vi "Module Loop.vi"(8 "error in (no error)":errorcluster, 11 "Debug GUI Module in":refnum<class "Debug GUI Module.lvclass">) -> (0 "error out":errorcluster, 3 "Debug GUI Module out":refnum<class "Debug GUI Module.lvclass">)   [LabVIEW 2020, in "VolatusGUI.lvlib" / "Debug GUI Module.lvclass"]
uses:
  Debug GUI Module.lvclass
  C:/dev/lv20CE/relink/lv-volatus/Volatus/Module/Module.lvclass
  Volatus/Module/Module.lvclass/Module.ctl
  Debug GUI Module.lvclass/Debug GUI Module.ctl
  Volatus/Module/Module.lvclass
  Show Module Data.ctl
  Volatus/Module Identity/Module Identity.lvclass/Module Identity.ctl
  Volatus/Show GUI Options.ctl
  Volatus/MessageQ/MessageQ.lvclass/MessageQ.ctl
  Volatus/Volatus Core Identity/Volatus Core Identity.lvclass
  C:/dev/lv20CE/relink/lv-volatus/Volatus/Identity/Identity.lvclass
  GUI Info.ctl
  Volatus/Module Identity/Module Identity.lvclass
  <vilib>/Utility/error.llb/Error Cluster From Error Code.vi
  Volatus/MessageQ/MessageQ.lvclass
  Volatus/VolatusAPI/VolatusAPI.lvclass
  Volatus/Volatus.lvlib
  GUI Helper/GUI Helper.lvclass
  VolatusGUI.lvlib
panel:
  in  "Show Metrics":bool
  in  "Modules":string(tree)
  out "Right-Click Info":string
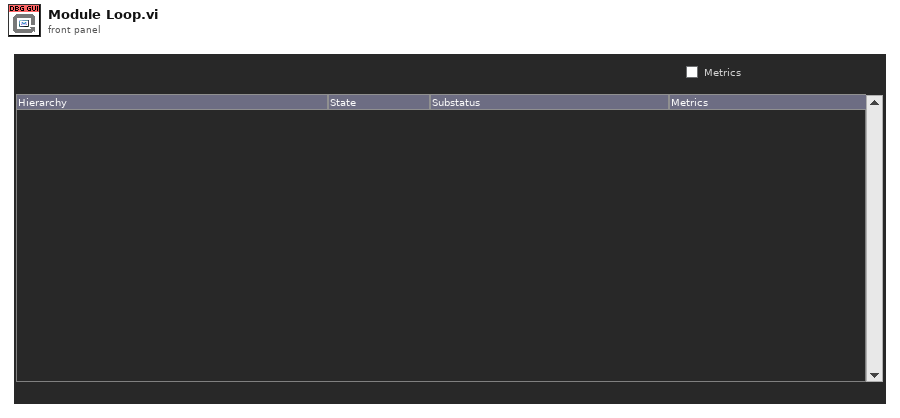
[diagram p1: front panel]
types:
  T1 = enum32{"Invalid", "Standard", "Closed", "Hidden", "Minimized", "Maximized"}
  T2 = typedef "VolatusGUI.lvlib/Show Module Data.ctl" = cluster{"ID":string, "BD":bool}
  T3 = typedef "Volatus.lvlib/Show GUI Options.ctl" = cluster{"Show Core Module":bool}
  T4 = typedef "VolatusGUI.lvlib/GUI Info.ctl" = cluster{"Color":u32, "Name":string}
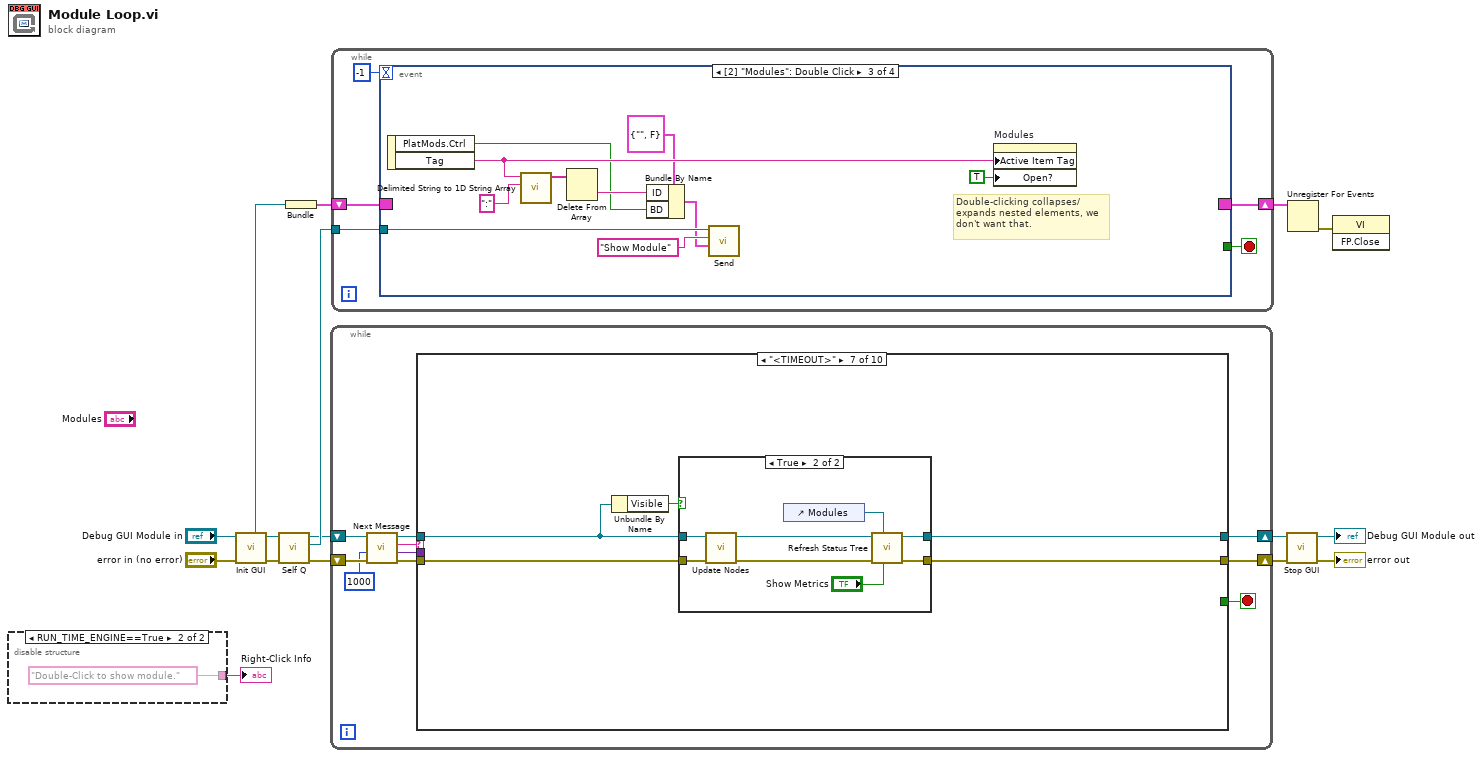
[diagram p0: block diagram]
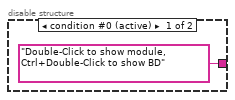
[diagram p2: hidden frame]
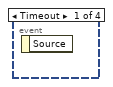
[diagram p3: hidden frame]
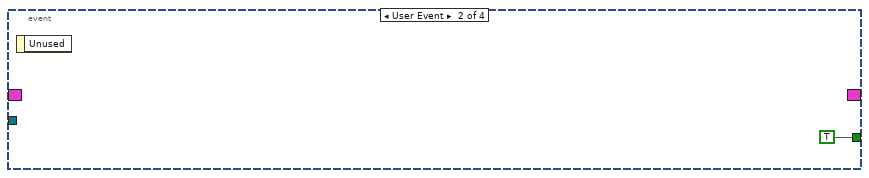
[diagram p4: hidden frame]
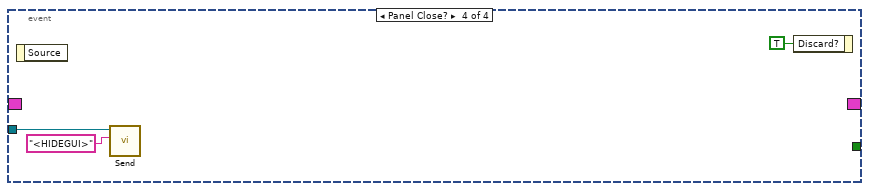
[diagram p5: hidden frame]
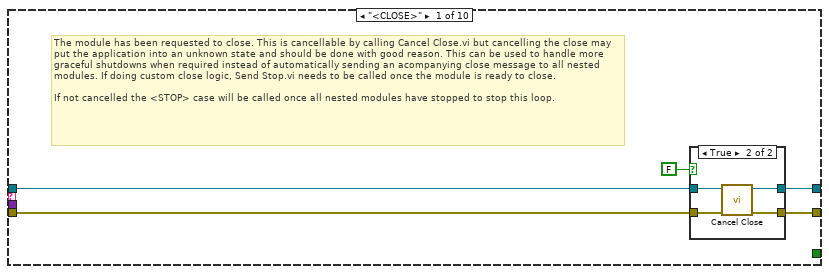
[diagram p6: hidden frame]
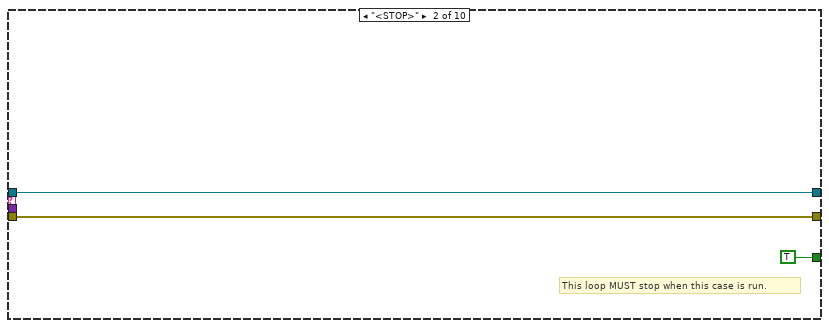
[diagram p8: hidden frame]
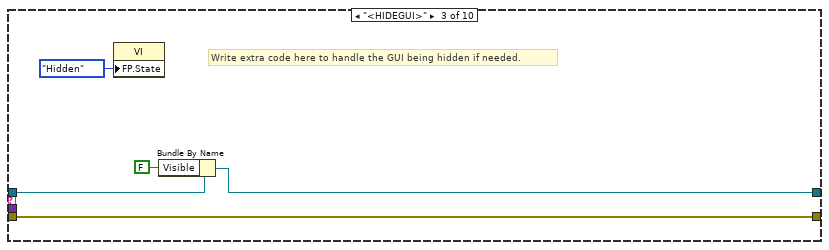
[diagram p9: hidden frame]
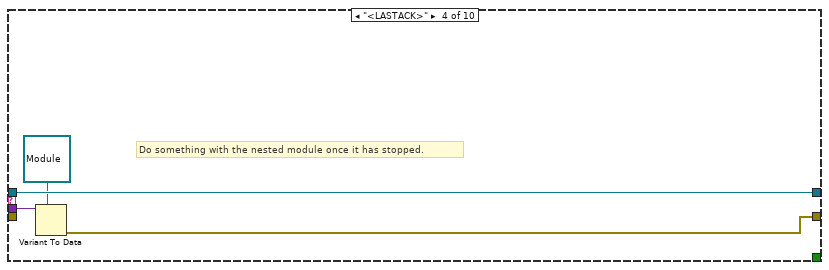
[diagram p10: hidden frame]
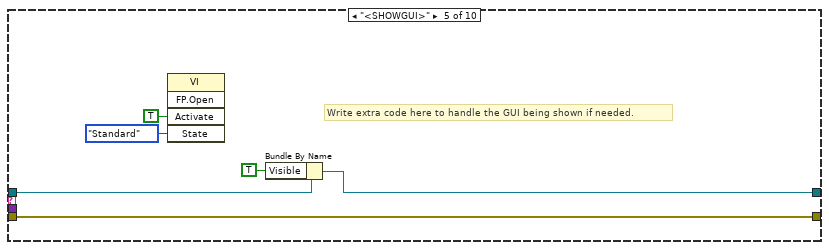
[diagram p11: hidden frame]
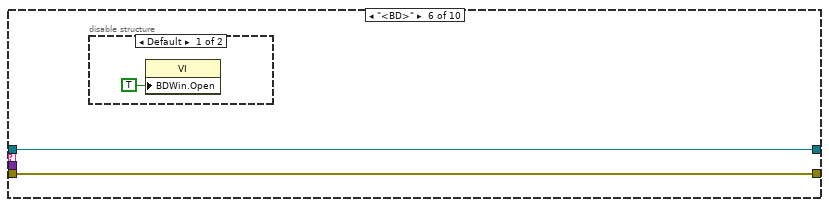
[diagram p12: hidden frame]
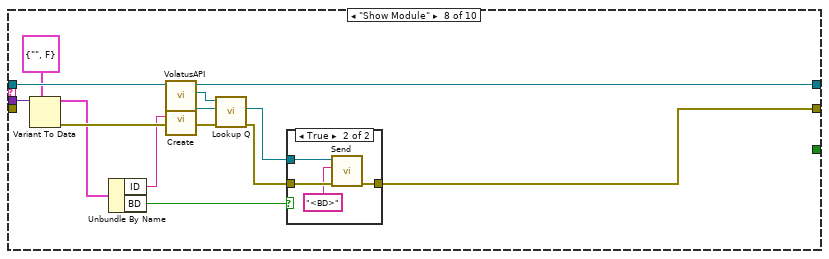
[diagram p15: hidden frame]
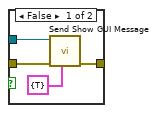
[diagram p16: hidden frame]
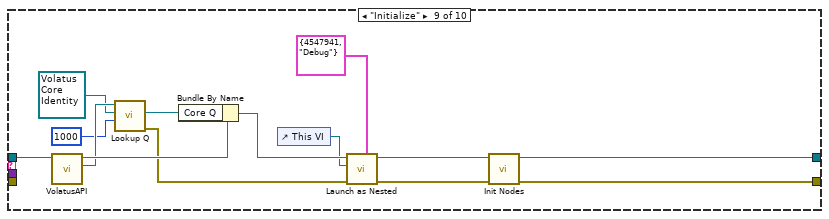
[diagram p17: hidden frame]
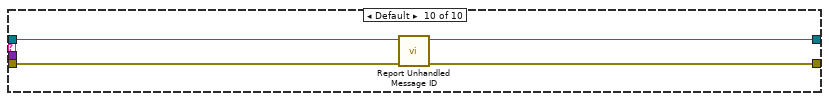
[diagram p18: hidden frame]
diagram:
  n1 = disable-structure shown="RUN_TIME_ENGINE==True" {
    disable-tunnel: ["Double-Click to show module, Ctrl+Double-Click to show BD" ("Right-Click Info") "Double-Click to show module." ("Right-Click Info")] -> w1
    frame condition #0 (active) {
    }
    frame condition #1 {
    }
  }
  "Right-Click Info" <- w1
  n2 = call "Init GUI.vi"("Module in"="Debug GUI Module in") -> ("Module out"=w8:refnum<class "Debug GUI Module.lvclass">, "Event Reg"=w13:refnum<event-registration>)  [unwired: 9 in]
  n3 = call "Self Q.vi"("Module in"=w8) -> ("Self Q"=w7:refnum<class "MessageQ.lvclass">, "Module out"=w6:refnum<class "Debug GUI Module.lvclass">)  [unwired: 9 in]
  n4 = Bundle("Event Reg"=w13) -> (w9:cluster{"Event Reg":refnum<event-registration>})  [unwired: 1 in]
  n5 = while {
    shift-right: [w21] -> w11
    shift-left: w6 -> [w26]
    shift-right: [w20] -> w12
    shift-left: "error in (no error)" -> [w25]
    stop <- w19 stop-if-true
    n6 = call "Next Message.vi"("error in (no error)"=w25, "Timeout ms (-1)"=1000, "Module in"=w26) -> ("error out"=w24:errorcluster, "Data"=w18:variant, "ID"=w23:string, "Module out"=w22:refnum<class "Debug GUI Module.lvclass">)  [unwired: 5 in]
    n7 = case shown="\"<TIMEOUT>\"" w23 {
      tunnel: w24 -> [w29 w39 w44 _ w54 w56 w63 _ _ w112]
      tunnel: w22 -> [w30 w40 w45 w49 w55 w57 w60 w86 w108 w110]
      tunnel: [w28 w40 w42 w49 w51 w57 w61 w84 w96 w109] -> w21
      tunnel: [w27 w39 w44 w46 w54 w56 w62 w78 w98 w111] -> w20
      tunnel: [_ TRUE _ _ _ _ _ _ _ _] -> w19
      tunnel: w18 -> [_ _ _ w48 _ _ _ w85 _ _]
      frame "<CLOSE>" {
        # "The module has been requested to close. This is cancellable by calling Cancel Close.vi but cancelling the close may put the application into an unknown state and should be done with good reason. This can be used to handle more graceful shutdowns when required instead of automatically sending an acompanying close message to all nested modules. If doing custom close logic, Send Stop.vi needs to be called once the module is ready to close.\n\nIf not cancelled the <STOP> case will be called once all nested modules have stopped to stop this loop."
        n8 = case shown="True" FALSE {
          tunnel: w29 -> [w32 w37]
          tunnel: [w32 w36] -> w27
          tunnel: w30 -> [w33 w35]
          tunnel: [w33 w34] -> w28
          frame False {
          }
          frame True {
            n9 = call "Cancel Close.vi"("error in (no error)"=w37, "Module in"=w35) -> ("error out"=w36:errorcluster, "Module out"=w34:refnum<class "Debug GUI Module.lvclass">)  [unwired: 8 in]
          }
        }
      }
      frame "<STOP>" {
        # "This loop MUST stop when this case is run."
      }
      frame "<HIDEGUI>" {
        # "Write extra code here to handle the GUI being hidden if needed."
        n10 = property class="VI"("FP.State"=T1."Hidden" ("Front Panel Window:State")) -> ()  [unwired: 2 in, 2 out]
        n11 = Bundle By Name(cluster=w45, "Visible"=FALSE) -> (w42:refnum<class "Debug GUI Module.lvclass">)
      }
      frame "<LASTACK>" {
        # "Do something with the nested module once it has stopped."
        n12 = Variant To Data(type=refnum<class "Module.lvclass"> refnum ("Volatus:Module"), Variant=w48) -> (error out=w46:errorcluster)  [unwired: 1 in, 1 out]
      }
      frame "<SHOWGUI>" {
        # "Write extra code here to handle the GUI being shown if needed."
        n13 = invoke class="VI" method="FP.Open"("Activate"=TRUE ("Activate?"), "State"=T1."Standard") -> ()  [unwired: 3 in, 5 out]
        n14 = Bundle By Name(cluster=w55, "Visible"=TRUE) -> (w51:refnum<class "Debug GUI Module.lvclass">)
      }
      frame "<BD>" {
        n15 = disable-structure shown="Default" {
          frame condition #0 (active) {
            n16 = property class="VI"("BDWin.Open"=TRUE ("Block Diagram Window:Open")) -> ()  [unwired: 2 in, 2 out]
          }
          frame condition #1 {
          }
        }
      }
      frame "<TIMEOUT>" {
        n17 = Unbundle By Name(w60) -> ("Visible"=w59:bool)
        n18 = case shown="True" w59 {
          tunnel: w63 -> [w64 w73]
          tunnel: [w64 w72] -> w62
          tunnel: [w65 w71] -> w61
          tunnel: w60 -> [w65 w68]
          frame False {
          }
          frame True {
            n19 = call "Update Nodes.vi"("error in (no error)"=w73, "Debug GUI Module in"=w68) -> ("error out"=w69:errorcluster, "Debug GUI Module out"=w67:refnum<class "Debug GUI Module.lvclass">)  [unwired: 8 in]
            n20 = control-ref of="Modules"() -> (w70:refnum<vi>)
            n21 = call "Refresh Status Tree.vi"("Show Metrics"="Show Metrics", "Tree Ref"=w70, "error in (no error)"=w69, "Debug GUI Module in"=w67) -> ("error out"=w72:errorcluster, "Debug GUI Module out"=w71:refnum<class "Debug GUI Module.lvclass">)  [unwired: 6 in]
          }
        }
      }
      frame "Show Module" {
        n22 = Variant To Data(type=T2 {"ID"="", "BD"=FALSE} ("Show Module Data"), Variant=w85) -> (data=w76:T2, error out=w81:errorcluster)  [unwired: 1 in]
        n23 = Unbundle By Name(w76) -> ("ID"=w75:string, "BD"=w74:bool)
        n24 = call "VolatusAPI.vi"("Module in"=w86) -> ("VolatusAPI"=w83:refnum<class "VolatusAPI.lvclass">, "Module out"=w84:refnum<class "Debug GUI Module.lvclass">)  [unwired: 9 in]
        n25 = call "Create.vi"("ID"=w75) -> ("Module Identity out"=w82:refnum<class "Module Identity.lvclass">)  [unwired: 10 in]
        n26 = call "Lookup Q.vi"("error in (no error)"=w81, "Identity"=w82, "VolatusAPI in"=w83) -> ("error out"=w79:errorcluster, "MessageQ"=w80:refnum<class "MessageQ.lvclass">)  [unwired: 6 in, 1 out]
        n27 = case shown="True" w74 {
          tunnel: w80 -> [w90 w93]
          tunnel: w79 -> [w89 w94]
          tunnel: [w87 w92] -> w78
          frame False {
            n28 = call "Send Show GUI Message.vi"("Show GUI Options"=T3 {"Show Core Module"=TRUE}, "error in (no error)"=w89, "MessageQ"=w90) -> ("error out"=w87:errorcluster)  [unwired: 8 in]
          }
          frame True {
            n29 = call "Send.vi"("error in (no error)"=w94, "ID"="<BD>", "MessageQ in"=w93) -> ("error out"=w92:errorcluster)  [unwired: 7 in, 1 out]
          }
        }
      }
      frame "Initialize" {
        n30 = call "VolatusAPI.vi"("Module in"=w108) -> ("VolatusAPI"=w106:refnum<class "VolatusAPI.lvclass">, "Module out"=w107:refnum<class "Debug GUI Module.lvclass">)  [unwired: 9 in]
        n31 = call "Lookup Q.vi"("Timeout ms (0)"=1000, "Identity"=refnum<class "Volatus Core Identity.lvclass"> refnum ("Volatus:Volatus Core Identity.lvclass"), "VolatusAPI in"=w106) -> ("error out"=w103:errorcluster, "MessageQ"=w104:refnum<class "MessageQ.lvclass">)  [unwired: 6 in, 1 out]
        n32 = Bundle By Name(cluster=w107, "Core Q"=w104) -> (w100:refnum<class "Debug GUI Module.lvclass">)
        n33 = control-ref of="This VI"() -> (w99:refnum<vi>)
        n34 = call "Launch as Nested.vi"("GUI Info (Default)"=T4 {"Color"=4547941, "Name"="Debug"}, "error in (no error)"=w103, "GUI"=w99, "Parent in"=w100) -> ("error out"=w101:errorcluster, "Parent"=w97:refnum<class "Debug GUI Module.lvclass">)  [unwired: 5 in, 1 out]
        n35 = call "Init Nodes.vi"("error in (no error)"=w101, "Debug GUI Module in"=w97) -> ("error out"=w98:errorcluster, "Debug GUI Module out"=w96:refnum<class "Debug GUI Module.lvclass">)  [unwired: 8 in]
      }
      frame Default {
        n36 = call "Report Unhandled Message ID.vi"("error in (no error)"=w112, "Module in"=w110) -> ("error out"=w111:errorcluster, "Module out"=w109:refnum<class "Debug GUI Module.lvclass">)  [unwired: 8 in]
      }
    }
  }
  n37 = while {
    tunnel: w7 -> [w117]
    shift-right: [w115] -> w10
    shift-left: w9 -> [w116]
    stop <- w114 stop-if-true
    n38 = event shown="[2] \"Modules\": Double Click" {
      selector: w116 -> [_ _ _ _]
      dyn-events: [_ _ _ _] -> w115
      timeout: -1 -> [_ _ _ _]
      tunnel: w117 -> [_ _ w126 w130]
      tunnel: [_ TRUE _ _] -> w114
      event Timeout {
        n39 = event-data() -> ()  [unwired: 1 in, 1 out]
      }
      event User Event {
        n40 = event-data() -> ()  [unwired: 1 in, 1 out]
      }
      event "Modules": Double Click {
        # "Double-clicking collapses/expands nested elements, we don't want that."
        n41 = event-data() -> ("PlatMods.Ctrl"=w120:bool, "Tag"=w124:string)  [unwired: 1 in]
        n42 = call <vilib>:"Delimited String to 1D String Array.vi"("delimiter"=":", "delimited string"=w124) -> ("string array"=w127:string[])  [unwired: 9 in]
        n43 = Delete From Array(array=w127) -> (deleted portion=w121:string)  [unwired: 2 in, 1 out]
        n44 = Bundle By Name(cluster=T2 {"ID"="", "BD"=FALSE} ("Show Module Data"), "ID"=w121, "BD"=w120) -> (w119:T2)
        n45 = call "Send.vi"("Data"=w119, "ID"="Show Module", "MessageQ in"=w126) -> ()  [unwired: 7 in, 2 out]
        n46 = property on="Modules" class="Tree (strict)"("Active Item Tag"=w124, "Open?"=TRUE ("Active Item:Open?")) -> ()  [unwired: 2 in, 2 out]
      }
      event Panel Close? {
        n47 = event-data() -> ()  [unwired: 1 in, 1 out]
        n48 = call "Send.vi"("ID"="<HIDEGUI>", "MessageQ in"=w130) -> ()  [unwired: 8 in, 2 out]
        n49 = event-data("Discard?"=TRUE) -> ()  [unwired: 1 in, 1 out]
      }
    }
  }
  n50 = call "Stop GUI.vi"("error in (no error)"=w12, "Module in"=w11) -> ("error out"=→"error out":errorcluster, "Module out"=→"Debug GUI Module out":refnum<class "Debug GUI Module.lvclass">)  [unwired: 8 in]
  n51 = Unregister For Events(event registration refnum=w10) -> (error out=w14:errorcluster)  [unwired: 1 in]
  n52 = invoke class="VI" method="FP.Close"(error in=w14) -> ()  [unwired: 2 in, 3 out]
